vi "test-linear-system-id.vi"(8 "error in (no error)":errorcluster) -> (0 "error out":errorcluster, 3 "All tests passed":bool)   [LabVIEW 2019]
uses:
  <vilib>/Rock Robotics/WPI/ThirdParty/JAS_Junk/TrajLib/LINEAR_SYSTEM.ctl
  <vilib>/Analysis/Matrix/Datatypes/RealMatrix.ctl
  <vilib>/Rock Robotics/WPI/ThirdParty/JAS_Junk/TrajLib/MatBuilder_Create.vi
  <vilib>/Rock Robotics/WPI/ThirdParty/JAS_Junk/TrajLib/MatrixHelper_Zero.vi
  <vilib>/Rock Robotics/WPI/ThirdParty/JAS_Junk/TrajLib/DCMotor_New.vi
  <vilib>/Rock Robotics/WPI/ThirdParty/JAS_Junk/TrajLib/Units_RotationsPerMinuteToRadiansPerSecond.vi
  <vilib>/Rock Robotics/WPI/ThirdParty/JAS_Junk/TrajLib/Matrix_Ident.vi
  <vilib>/Rock Robotics/WPI/ThirdParty/JAS_Junk/TrajLib/LinearSystem_New.vi
  <vilib>/Analysis/7linalg.llb/Create Special Matrix.vi
  <vilib>/Analysis/7linalg.llb/Create Special Real Matrix.vi
  <vilib>/Rock Robotics/WPI/ThirdParty/JAS_Junk/TrajLib/Trajectory_Library.lvlib
  <vilib>/Analysis/Matrix/NI_Matrix.lvlib
panel:
  out "T B 5":bool
  out "T A 5":bool
  out "T B 4":bool
  out "T A 4":bool
  out "T D 3":bool
  out "T C 3":bool
  out "T B 3":bool
  out "T A 3":bool
  out "T D 2":bool
  out "T C 2":bool
  out "T B 2":bool
  out "T A 2":bool
  out "T D 1":bool
  out "T C 1":bool
  out "T B 1":bool
  out "T A 1":bool
  out "IdentifyVelocitySystem":T1
  out "IdentifyPositionSystem":T1
  out "FlyWheel":T1
  out "DriveTrain":T1
  out "Elevator":T1
  # "A  = -10.14132, 3.06598, \n            3.06598, -10.14132\n\nB =    4.2590,   -1.28762, \n         -1.2876,   4.2590\n\nC =   1.0,   0.0, \n          0.0,  1.0;\n\nD =   0.0,   0.0, \n          0.0,   0.0"
  # "A   = (0, 1, \n               0, -99.05473)\n\n     B = (0, \n            20.8)\n\n   C   = 1, 0\n\n    D = 0"
  # "A = -26.87032\n\nB = 1354.166667;\n\nC = 1\n\nD = 0"
  # "A =   0, 1, \n         0, -1 / 0.5\n\nB =  0, \n        1 / 0.5"
  # "A =   -1.0 / 0.5\n\nB = 1 / 0.5"
  # "<States,States>"
  # "<States,Inputs>"
  # "<Outputs,States>"
  # "<Outputs,Inputs>"
  # "<States,States>"
  # "<States,Inputs>"
  # "<Outputs,States>"
  # "<Outputs,Inputs>"
  # "<States,States>"
  # "<States,Inputs>"
  # "<Outputs,States>"
  # "<Outputs,Inputs>"
  # "<States,States>"
  # "<States,Inputs>"
  # "<Outputs,States>"
  # "<Outputs,Inputs>"
  # "<States,States>"
  # "<States,Inputs>"
  # "<Outputs,States>"
  # "<Outputs,Inputs>"
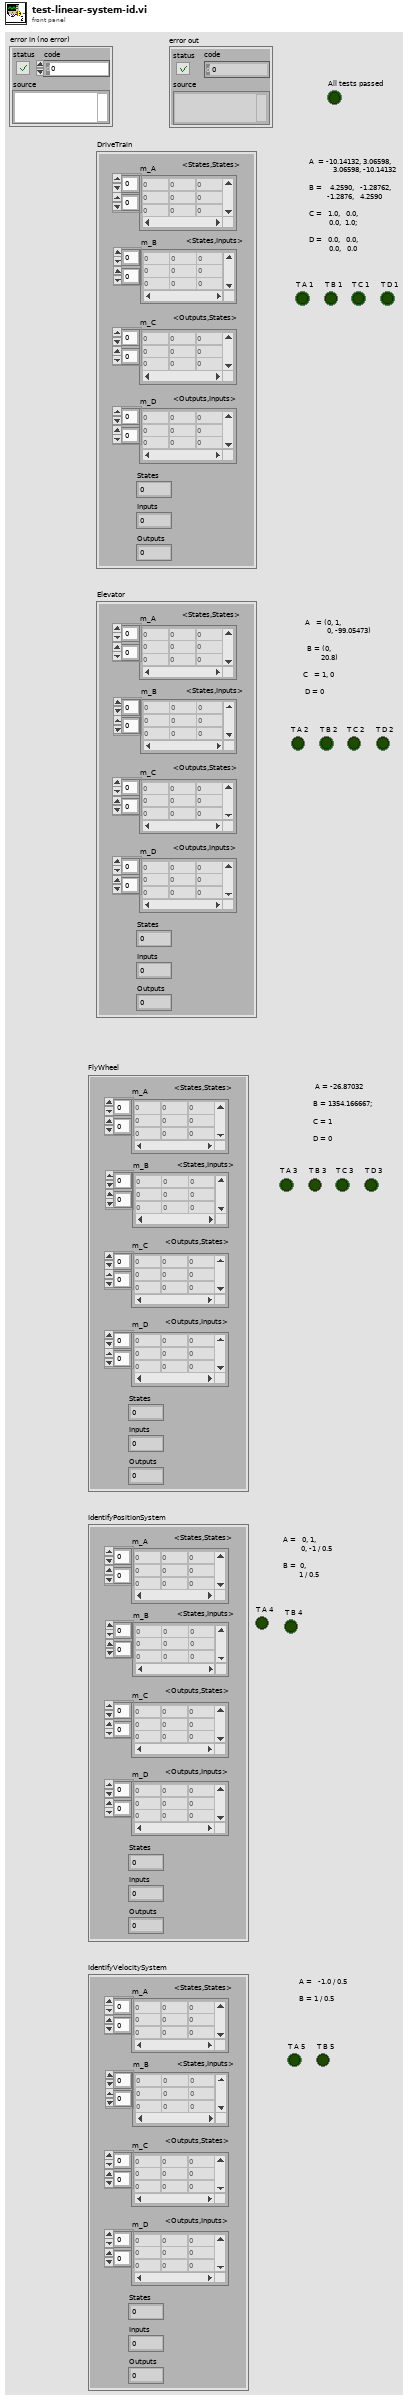
[diagram p1: front panel]
types:
  T1 = typedef "Trajectory_Library.lvlib/LINEAR_SYSTEM.ctl" = cluster{"m_A":T2, "m_B":T2, "m_C":T2, "m_D":T2, "States":i32, "Inputs":i32, "Outputs":i32}
  T2 = typedef "NI_Matrix.lvlib/RealMatrix.ctl" = dbl[][]
  T3 = typedef "Trajectory_Library.lvlib/DCMOTOR.CTL" = cluster{"nominalVoltage_Volts":dbl, "StallTorque_NM":dbl, "StallCurrent_Amps":dbl, "FreeCurrent_Amps":dbl, "FreeSpeed_RadPerSec":dbl, "R_Ohms":dbl, "KvINV_RadPerSecPerVolt":dbl, "Kt_NMPerAmp":dbl, "L_H":dbl, "Jr_KgM2":dbl}
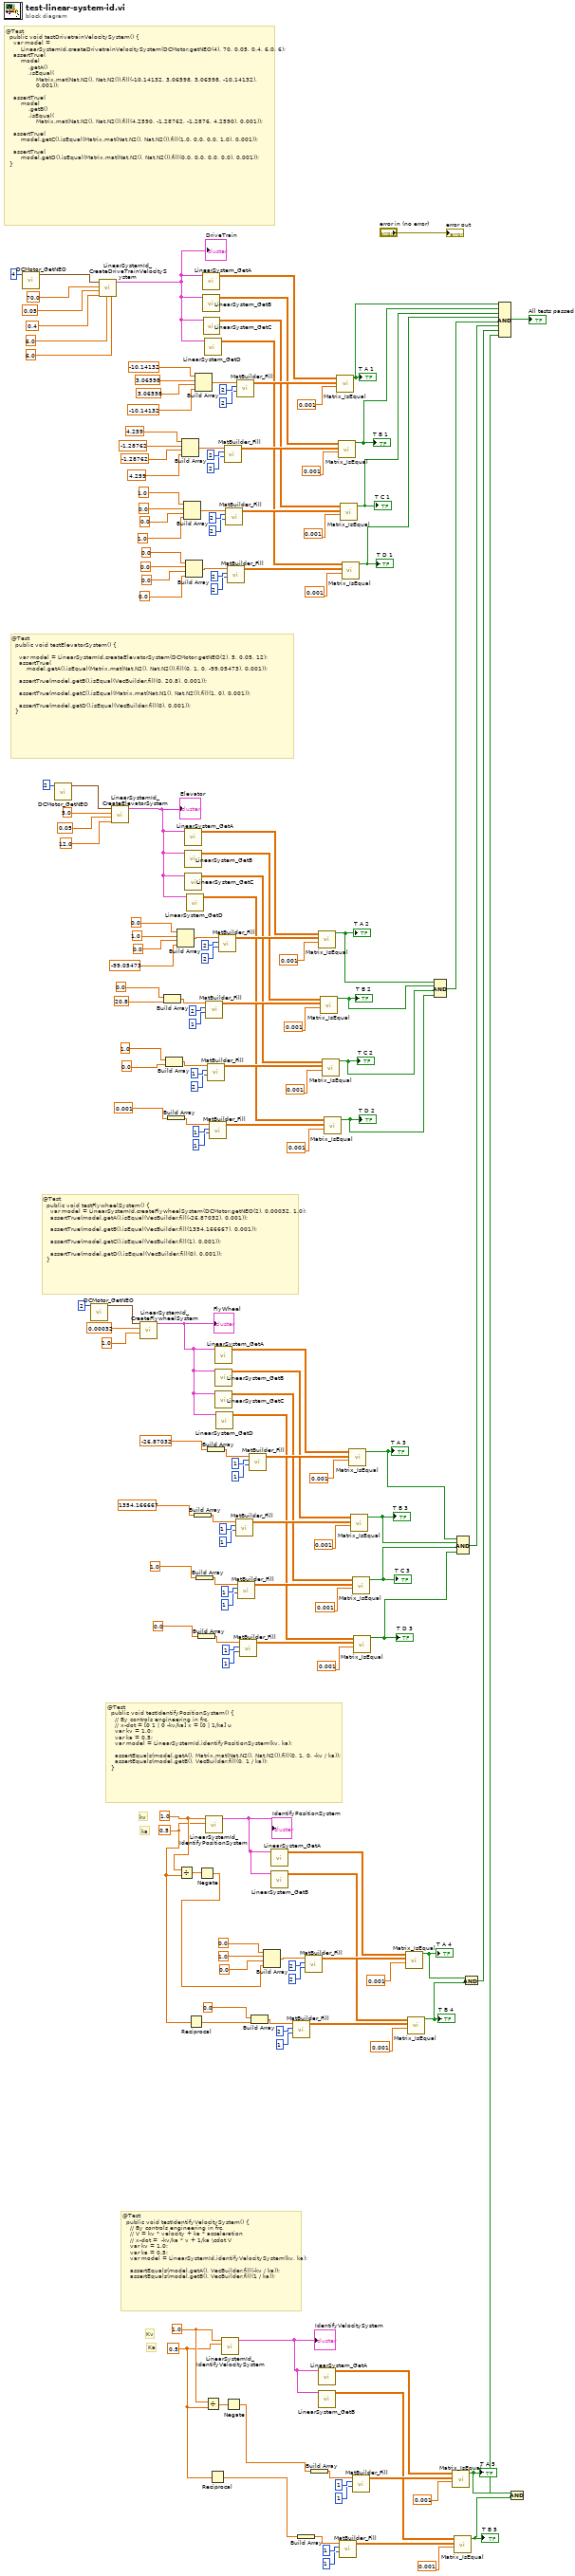
[diagram p0: block diagram]
diagram:
  w25 = 0.5 ("kA")
  w27 = 1.0 ("kV")
  w29 = 0.5 ("kA")
  w32 = 1.0 ("kV")
  # "Ka"
  # "Kv"
  # "ka"
  # "kv"
  # "@Test\n  public void testIdentifyVelocitySystem() {\n    // By controls engineering in frc,\n    // V = kv * velocity + ka * acceleration\n    // x-dot =  -kv/ka * v + 1/ka \\cdot V\n    var kv = 1.0;\n    var ka = 0.5;\n    var model = LinearSystemId.identifyVelocitySystem(kv, ka);\n\n    assertEquals(model.getA(), VecBuilder.fill(-kv / ka));\n    assertEquals(model.getB(), VecBuilder.fill(1 / ka));"
  # "@Test\n  public void testIdentifyPositionSystem() {\n    // By controls engineering in frc,\n    // x-dot = [0 1 | 0 -kv/ka] x = [0 | 1/ka] u\n    var kv = 1.0;\n    var ka = 0.5;\n    var model = LinearSystemId.identifyPositionSystem(kv, ka);\n\n    assertEquals(model.getA(), Matrix.mat(Nat.N2(), Nat.N2()).fill(0, 1, 0, -kv / ka));\n    assertEquals(model.getB(), VecBuilder.fill(0, 1 / ka));\n  }"
  # "@Test\n  public void testFlywheelSystem() {\n    var model = LinearSystemId.createFlywheelSystem(DCMotor.getNEO(2), 0.00032, 1.0);\n    assertTrue(model.getA().isEqual(VecBuilder.fill(-26.87032), 0.001));\n\n    assertTrue(model.getB().isEqual(VecBuilder.fill(1354.166667), 0.001));\n\n    assertTrue(model.getC().isEqual(VecBuilder.fill(1), 0.001));\n\n    assertTrue(model.getD().isEqual(VecBuilder.fill(0), 0.001));\n  }"
  # "@Test\n  public void testDrivetrainVelocitySystem() {\n    var model =\n        LinearSystemId.createDrivetrainVelocitySystem(DCMotor.getNEO(4), 70, 0.05, 0.4, 6.0, 6);\n    assertTrue(\n        model\n            .getA()\n            .isEqual(\n                Matrix.mat(Nat.N2(), Nat.N2()).fill(-10.14132, 3.06598, 3.06598, -10.14132),\n                0.001));\n\n    assertTrue(\n        model\n            .getB()\n            .isEqual(\n                Matrix.mat(Nat.N2(), Nat.N2()).fill(4.2590, -1.28762, -1.2876, 4.2590), 0.001));\n\n    assertTrue(\n        model.getC().isEqual(Matrix.mat(Nat.N2(), Nat.N2()).fill(1.0, 0.0, 0.0, 1.0), 0.001));\n\n    assertTrue(\n        model.getD().isEqual(Matrix.mat(Nat.N2(), Nat.N2()).fill(0.0, 0.0, 0.0, 0.0), 0.001));\n  }"
  # "@Test\n  public void testElevatorSystem() {\n\n    var model = LinearSystemId.createElevatorSystem(DCMotor.getNEO(2), 5, 0.05, 12);\n    assertTrue(\n        model.getA().isEqual(Matrix.mat(Nat.N2(), Nat.N2()).fill(0, 1, 0, -99.05473), 0.001));\n\n    assertTrue(model.getB().isEqual(VecBuilder.fill(0, 20.8), 0.001));\n\n    assertTrue(model.getC().isEqual(Matrix.mat(Nat.N1(), Nat.N2()).fill(1, 0), 0.001));\n\n    assertTrue(model.getD().isEqual(VecBuilder.fill(0), 0.001));\n  }"
  n1 = call <vilib>:"DCMotor_GetNEO.vi"("Num Motors"=4) -> ("DCMOTOR"=w176:T3)  [unwired: 10 in]
  n2 = call <vilib>:"DCMotor_GetNEO.vi"("Num Motors"=2) -> ("DCMOTOR"=w181:T3)  [unwired: 10 in]
  n3 = call <vilib>:"DCMotor_GetNEO.vi"("Num Motors"=2) -> ("DCMOTOR"=w169:T3)  [unwired: 10 in]
  n4 = call <vilib>:"LinearSystemId_CreateDriveTrainVelocitySystem.vi"("G"=6.0, "JKgMetersSquared"=6.0, "rbMeters"=0.4, "rMeters"=0.05, "MassKg"=70.0, "Motor"=w176) -> ("Linearsystem"=w146:T1)  [unwired: 4 in, 1 out]
  "DriveTrain" <- w146
  n5 = call <vilib>:"LinearSystemId_CreateElevatorSystem.vi"("G"=12.0, "radiusMeters"=0.05, "massKg"=5.0, "DCMOTOR"=w181) -> ("Linearsystem"=w93:T1)  [unwired: 6 in, 1 out]
  "Elevator" <- w93
  n6 = call <vilib>:"LinearSystemId_CreateFlywheelSystem.vi"("G"=1.0, "jKgMetersSquared"=0.00032, "DCMOTOR"=w169) -> ("Linearsystem"=w64:T1)  [unwired: 7 in, 1 out]
  "FlyWheel" <- w64
  n7 = Build Array(0.0 ("element"), 20.8 ("element")) -> (w115:dbl[])
  n8 = Build Array(1.0 ("element"), 0.0 ("element")) -> (w107:dbl[])
  n9 = Build Array(0.001 ("element")) -> (w101:dbl[])
  n10 = Build Array(0.0 ("element"), 1.0 ("element"), 0.0 ("element"), -99.05473 ("element")) -> (w125:dbl[])
  n11 = Divide(x=w32, y=w29) -> (x/y=w33:dbl)
  n12 = Build Array(4.259 ("element"), -1.28762 ("element"), -1.28762 ("element"), 4.259 ("element")) -> (w156:dbl[])
  n13 = Build Array(1.0 ("element"), 0.0 ("element"), 0.0 ("element"), 1.0 ("element")) -> (w145:dbl[])
  n14 = call <vilib>:"LinearSystem_GetA.vi"("Linearsystem"=w93) -> ("A"=w118:T2)  [unwired: 10 in]
  n15 = call <vilib>:"LinearSystem_GetB.vi"("Linearsystem"=w93) -> ("B"=w108:T2)  [unwired: 10 in]
  n16 = call <vilib>:"LinearSystem_GetC.vi"("Linearsystem"=w93) -> ("C"=w95:T2)  [unwired: 10 in]
  n17 = Build Array(0.0 ("element"), 0.0 ("element"), 0.0 ("element"), 0.0 ("element")) -> (w136:dbl[])
  n18 = call <vilib>:"LinearSystem_GetD.vi"("Linearsystem"=w93) -> ("D"=w94:T2)  [unwired: 10 in]
  n19 = Reciprocal(x=w29) -> (1/x=w30:dbl)
  n20 = Build Array(1354.166667 ("element")) -> (w85:dbl[])
  n21 = Build Array(-10.14132 ("element"), 3.06598 ("element"), 3.06598 ("element"), -10.14132 ("element")) -> (w166:dbl[])
  n22 = Build Array(1.0 ("element")) -> (w78:dbl[])
  n23 = Build Array(0.0 ("element")) -> (w72:dbl[])
  n24 = Negate(x=w33) -> (-x=w31:dbl)
  n25 = call <vilib>:"LinearSystem_GetA.vi"("Linearsystem"=w146) -> ("A"=w159:T2)  [unwired: 10 in]
  n26 = call <vilib>:"LinearSystem_GetB.vi"("Linearsystem"=w146) -> ("B"=w147:T2)  [unwired: 10 in]
  n27 = call <vilib>:"LinearSystem_GetC.vi"("Linearsystem"=w146) -> ("C"=w127:T2)  [unwired: 10 in]
  n28 = call <vilib>:"LinearSystem_GetD.vi"("Linearsystem"=w146) -> ("D"=w126:T2)  [unwired: 10 in]
  n29 = Divide(x=w27, y=w25) -> (x/y=w28:dbl)
  n30 = call <vilib>:"LinearSystemId_IdentifyPositionSystem.vi"("kA"=w29, "kV"=w32) -> ("Linearsystem"=w47:T1)  [unwired: 8 in, 1 out]
  "IdentifyPositionSystem" <- w47
  n31 = call <vilib>:"MatBuilder_Fill.vi"("Columns"=1, "Rows"=2, "Value List"=w115) -> ("output matrix"=w110:T2)  [unwired: 8 in]
  n32 = Build Array(-26.87032 ("element")) -> (w92:dbl[])
  n33 = call <vilib>:"MatBuilder_Fill.vi"("Columns"=2, "Rows"=1, "Value List"=w107) -> ("output matrix"=w103:T2)  [unwired: 8 in]
  n34 = call <vilib>:"MatBuilder_Fill.vi"("Columns"=1, "Rows"=1, "Value List"=w101) -> ("output matrix"=w97:T2)  [unwired: 8 in]
  n35 = Reciprocal(x=w25) -> (1/x=w23:dbl)
  n36 = call <vilib>:"LinearSystem_GetA.vi"("Linearsystem"=w64) -> ("A"=w88:T2)  [unwired: 10 in]
  n37 = call <vilib>:"LinearSystem_GetB.vi"("Linearsystem"=w64) -> ("B"=w79:T2)  [unwired: 10 in]
  n38 = call <vilib>:"LinearSystem_GetC.vi"("Linearsystem"=w64) -> ("C"=w66:T2)  [unwired: 10 in]
  n39 = call <vilib>:"LinearSystem_GetD.vi"("Linearsystem"=w64) -> ("D"=w65:T2)  [unwired: 10 in]
  n40 = call <vilib>:"MatBuilder_Fill.vi"("Columns"=2, "Rows"=2, "Value List"=w125) -> ("output matrix"=w117:T2)  [unwired: 8 in]
  n41 = call <vilib>:"LinearSystemId_IdentifyVelocitySystem.vi"("kA"=w25, "kV"=w27) -> ("Linearsystem"=w35:T1)  [unwired: 8 in, 1 out]
  "IdentifyVelocitySystem" <- w35
  n42 = call <vilib>:"MatBuilder_Fill.vi"("Columns"=2, "Rows"=2, "Value List"=w156) -> ("output matrix"=w149:T2)  [unwired: 8 in]
  n43 = Negate(x=w28) -> (-x=w26:dbl)
  n44 = call <vilib>:"MatBuilder_Fill.vi"("Columns"=2, "Rows"=2, "Value List"=w145) -> ("output matrix"=w138:T2)  [unwired: 8 in]
  n45 = call <vilib>:"MatBuilder_Fill.vi"("Columns"=2, "Rows"=2, "Value List"=w136) -> ("output matrix"=w129:T2)  [unwired: 8 in]
  n46 = call <vilib>:"MatBuilder_Fill.vi"("Columns"=1, "Rows"=1, "Value List"=w85) -> ("output matrix"=w81:T2)  [unwired: 8 in]
  n47 = call <vilib>:"MatBuilder_Fill.vi"("Columns"=2, "Rows"=2, "Value List"=w166) -> ("output matrix"=w158:T2)  [unwired: 8 in]
  n48 = call <vilib>:"MatBuilder_Fill.vi"("Columns"=1, "Rows"=1, "Value List"=w78) -> ("output matrix"=w74:T2)  [unwired: 8 in]
  n49 = call <vilib>:"MatBuilder_Fill.vi"("Columns"=1, "Rows"=1, "Value List"=w72) -> ("output matrix"=w68:T2)  [unwired: 8 in]
  n50 = call <vilib>:"MatBuilder_Fill.vi"("Columns"=1, "Rows"=1, "Value List"=w92) -> ("output matrix"=w87:T2)  [unwired: 8 in]
  n51 = Build Array(0.0 ("element"), w30) -> (w54:dbl[])
  n52 = Build Array(0.0 ("element"), 1.0 ("element"), 0.0 ("element"), w31) -> (w63:dbl[])
  n53 = call <vilib>:"LinearSystem_GetA.vi"("Linearsystem"=w47) -> ("A"=w57:T2)  [unwired: 10 in]
  n54 = call <vilib>:"LinearSystem_GetB.vi"("Linearsystem"=w47) -> ("B"=w48:T2)  [unwired: 10 in]
  n55 = call <vilib>:"MatBuilder_Fill.vi"("Columns"=1, "Rows"=2, "Value List"=w54) -> ("output matrix"=w50:T2)  [unwired: 8 in]
  n56 = Build Array(w23) -> (w24:dbl[])
  n57 = call <vilib>:"MatBuilder_Fill.vi"("Columns"=2, "Rows"=2, "Value List"=w63) -> ("output matrix"=w56:T2)  [unwired: 8 in]
  n58 = Build Array(w26) -> (w46:dbl[])
  n59 = call <vilib>:"LinearSystem_GetA.vi"("Linearsystem"=w35) -> ("A"=w43:T2)  [unwired: 10 in]
  n60 = call <vilib>:"LinearSystem_GetB.vi"("Linearsystem"=w35) -> ("B"=w36:T2)  [unwired: 10 in]
  n61 = call <vilib>:"Matrix_IsEqual.vi"("Tolerance"=0.001, "other"=w117, "input matrix"=w118) -> ("Equal"=w17:bool)  [unwired: 8 in]
  "T A 2" <- w17
  n62 = call <vilib>:"Matrix_IsEqual.vi"("Tolerance"=0.001, "other"=w110, "input matrix"=w108) -> ("Equal"=w16:bool)  [unwired: 8 in]
  "T B 2" <- w16
  n63 = call <vilib>:"Matrix_IsEqual.vi"("Tolerance"=0.001, "other"=w103, "input matrix"=w95) -> ("Equal"=w15:bool)  [unwired: 8 in]
  "T C 2" <- w15
  n64 = call <vilib>:"Matrix_IsEqual.vi"("Tolerance"=0.001, "other"=w97, "input matrix"=w94) -> ("Equal"=w14:bool)  [unwired: 8 in]
  "T D 2" <- w14
  n65 = call <vilib>:"Matrix_IsEqual.vi"("Tolerance"=0.001, "other"=w158, "input matrix"=w159) -> ("Equal"=w21:bool)  [unwired: 8 in]
  "T A 1" <- w21
  n66 = call <vilib>:"Matrix_IsEqual.vi"("Tolerance"=0.001, "other"=w149, "input matrix"=w147) -> ("Equal"=w20:bool)  [unwired: 8 in]
  "T B 1" <- w20
  n67 = call <vilib>:"MatBuilder_Fill.vi"("Columns"=1, "Rows"=1, "Value List"=w24) -> ("output matrix"=w38:T2)  [unwired: 8 in]
  n68 = call <vilib>:"Matrix_IsEqual.vi"("Tolerance"=0.001, "other"=w138, "input matrix"=w127) -> ("Equal"=w19:bool)  [unwired: 8 in]
  "T C 1" <- w19
  n69 = call <vilib>:"Matrix_IsEqual.vi"("Tolerance"=0.001, "other"=w129, "input matrix"=w126) -> ("Equal"=w18:bool)  [unwired: 8 in]
  "T D 1" <- w18
  n70 = call <vilib>:"Matrix_IsEqual.vi"("Tolerance"=0.001, "other"=w87, "input matrix"=w88) -> ("Equal"=w12:bool)  [unwired: 8 in]
  "T A 3" <- w12
  n71 = call <vilib>:"Matrix_IsEqual.vi"("Tolerance"=0.001, "other"=w81, "input matrix"=w79) -> ("Equal"=w11:bool)  [unwired: 8 in]
  "T B 3" <- w11
  n72 = call <vilib>:"Matrix_IsEqual.vi"("Tolerance"=0.001, "other"=w74, "input matrix"=w66) -> ("Equal"=w10:bool)  [unwired: 8 in]
  "T C 3" <- w10
  n73 = call <vilib>:"MatBuilder_Fill.vi"("Columns"=1, "Rows"=1, "Value List"=w46) -> ("output matrix"=w42:T2)  [unwired: 8 in]
  n74 = call <vilib>:"Matrix_IsEqual.vi"("Tolerance"=0.001, "other"=w68, "input matrix"=w65) -> ("Equal"=w9:bool)  [unwired: 8 in]
  "T D 3" <- w9
  n75 = call <vilib>:"Matrix_IsEqual.vi"("Tolerance"=0.001, "other"=w56, "input matrix"=w57) -> ("Equal"=w7:bool)  [unwired: 8 in]
  "T A 4" <- w7
  n76 = call <vilib>:"Matrix_IsEqual.vi"("Tolerance"=0.001, "other"=w50, "input matrix"=w48) -> ("Equal"=w6:bool)  [unwired: 8 in]
  "T B 4" <- w6
  n77 = Compound Arithmetic op=AND(w17, w16, w15, w14) -> (w13:bool)
  n78 = call <vilib>:"Matrix_IsEqual.vi"("Tolerance"=0.001, "other"=w42, "input matrix"=w43) -> ("Equal"=w4:bool)  [unwired: 8 in]
  "T A 5" <- w4
  n79 = call <vilib>:"Matrix_IsEqual.vi"("Tolerance"=0.001, "other"=w38, "input matrix"=w36) -> ("Equal"=w3:bool)  [unwired: 8 in]
  "T B 5" <- w3
  n80 = Compound Arithmetic op=AND(w12, w11, w10, w9) -> (w8:bool)
  n81 = Compound Arithmetic op=AND(w7, w6) -> (w5:bool)
  n82 = Compound Arithmetic op=AND(w4, w3) -> (w2:bool)
  n83 = Compound Arithmetic op=AND(w21, w20, w19, w18, w13, w8, w5, w2) -> (→"All tests passed":bool)
  "error out" <- "error in (no error)"
